vi "Configure TEC.vi"(0 "VISA resource name":refnum<visa-resource-name>, 5 "Enable TEC (Enabled)":bool=TRUE, 7 "Enable Fan (Enabled)":bool=TRUE, 9 "TEC Setpoint Temperature (-5)":dbl=-5.0, 11 "error in (no error)":errorcluster) -> (4 "VISA resource name out":refnum<visa-resource-name>, 15 "error out":errorcluster)   [LabVIEW 2018, in "Ocean Optics 2000 4000.lvlib"]
doc: "Configures the Thermo Electric Cooling (TEC) settings such as enable TEC, enable Fan and also TEC Setpoint Temperature.\n\n<b>Note:</b>\nOnly applicable on NIRQuest512, NIRQuest256 and QE65000."
uses:
  Ocean Optics 2000 4000.lvlib
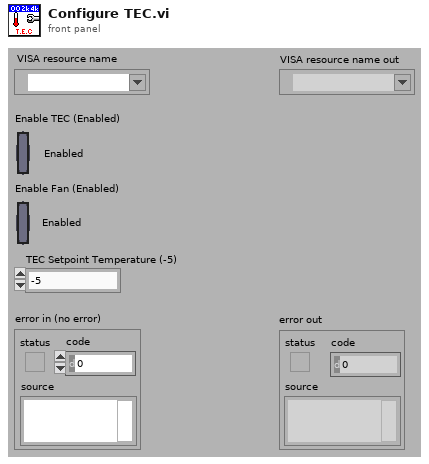
[diagram p1: front panel]
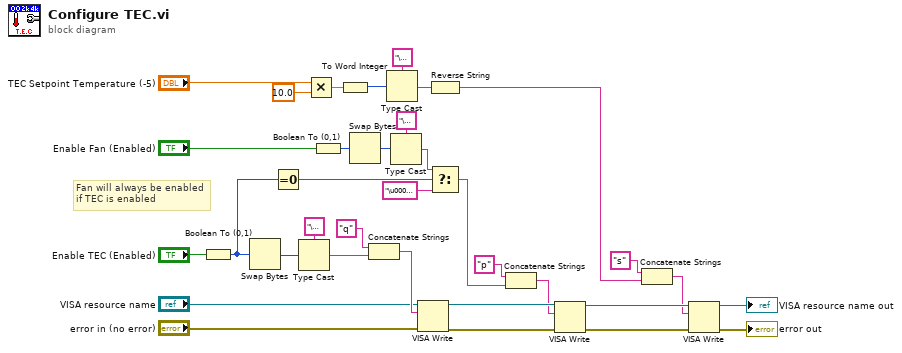
[diagram p0: block diagram]
diagram:
  # "Fan will always be enabled if TEC is enabled"
  n1 = Boolean To (0,1)(Boolean="Enable TEC (Enabled)") -> (0, 1=w26:i16)
  n2 = Swap Bytes(anything=w26) -> (byte swapped=w33:i16)
  n3 = Equal To 0?(x=w26) -> (x = 0?=w20:bool)
  n4 = Type Cast(type="\u0000", x=w33) -> (*(type *) &x=w31:string)
  n5 = Multiply(x="TEC Setpoint Temperature (-5)", y=10.0) -> (x*y=w12:dbl)
  n6 = Boolean To (0,1)(Boolean="Enable Fan (Enabled)") -> (0, 1=w22:i16)
  n7 = To Word Integer(number=w12) -> (16bit integer=w8:i16)
  n8 = Swap Bytes(anything=w22) -> (byte swapped=w21:i16)
  n9 = Concatenate Strings("q" ("string"), w31) -> (w29:string)
  n10 = Type Cast(type="\u0000", x=w8) -> (*(type *) &x=w7:string)
  n11 = Type Cast(type="\u0000", x=w21) -> (*(type *) &x=w19:string)
  n12 = VISA Write(VISA resource name="VISA resource name", write buffer=w29, error in (no error)="error in (no error)") -> (VISA resource name out=w16:refnum<visa-resource-name>, error out=w15:errorcluster)  [unwired: 1 out]
  n13 = Reverse String(1:w7) -> (0:w1:string)
  n14 = Select(t=w19, s=w20, f="\u0001\u0000") -> (s? t:f=w17:string)
  n15 = Concatenate Strings("p" ("string"), w17) -> (w11:string)
  n16 = VISA Write(VISA resource name=w16, write buffer=w11, error in (no error)=w15) -> (VISA resource name out=w10:refnum<visa-resource-name>, error out=w6:errorcluster)  [unwired: 1 out]
  n17 = Concatenate Strings("s" ("string"), w1) -> (w2:string)
  n18 = VISA Write(VISA resource name=w10, write buffer=w2, error in (no error)=w6) -> (VISA resource name out=→"VISA resource name out":refnum<visa-resource-name>, error out=→"error out":errorcluster)  [unwired: 1 out]
